vi "write_fifo_resonance_toggle_and_FF_FB.vi"(5 "enable fly-back reversion?":bool, 7 "fly-back?":bool, 8 "pixel finished?":bool, 9 "mark fly-back":bool=TRUE, 11 "integration cluster in":T1) -> (0 "FIFO overflow out":bool, 3 "integration cluster out":T1)   [LabVIEW 2010]
uses:
  integration_cluster.ctl
  <vilib>/rvi/DataTransferAndStorage/Container/XNode/niFpgaContainer.xnode
  <vilib>/rvi/DataTransferAndStorage/Container/Common/niFpgaContainerMethod.ctl
  <vilib>/rvi/DataTransferAndStorage/Container/Common/niFpgaTransferTypeControl.ctl
  <vilib>/rvi/Memory/Memory_Emulation/nirvimemoryEmulationManagerCache_GetValue.vi
  <vilib>/rvi/DataTransferAndStorage/Container/Common/niFpgaContainerGetUniqueNameForEmu.vi
  <vilib>/rvi/Memory/Memory_Emulation/nirvimemoryEmulationManagerCache_InsertValue.vi
  <vilib>/Utility/error.llb/Clear Errors.vi
  <vilib>/rvi/Memory/Memory_Emulation/nirvimemoryEmulationManagerCache_SetValue.vi
  <vilib>/rvi/interface/RandomDataEmulation/nirviRandomDataFPGAFIFO.vi
  <vilib>/rvi/interface/RandomDataEmulation/niFpgaRandomDataHandleErrors.vi
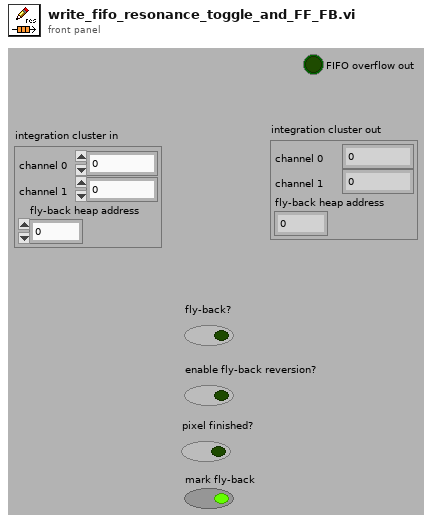
[diagram p1: front panel]
types:
  T1 = typedef "integration_cluster.ctl" = cluster{"channel 0":u32, "channel 1":u32, "fly-back heap address":u32}
  T2 = typedef "niFpgaContainerMethod.ctl" = enum16{"<none>", "write", "read", "clear", "getNumberOfElementsToWrite", "getNumberOfElementsToRead", "enable", "disable", "flushAndDisable", "getStreamState", "readA", "readB", "dramWrite", "dramWriteWithByteEnables", "dramRequestData", "dramRetrieveData"}
  T3 = typedef "niFpgaTransferTypeControl.ctl" = enum16{"Target-Scoped", "Host to Target - DMA", "Target to Host - DMA", "Peer to Peer Reader", "Peer to Peer Writer", "Bidirectional"}
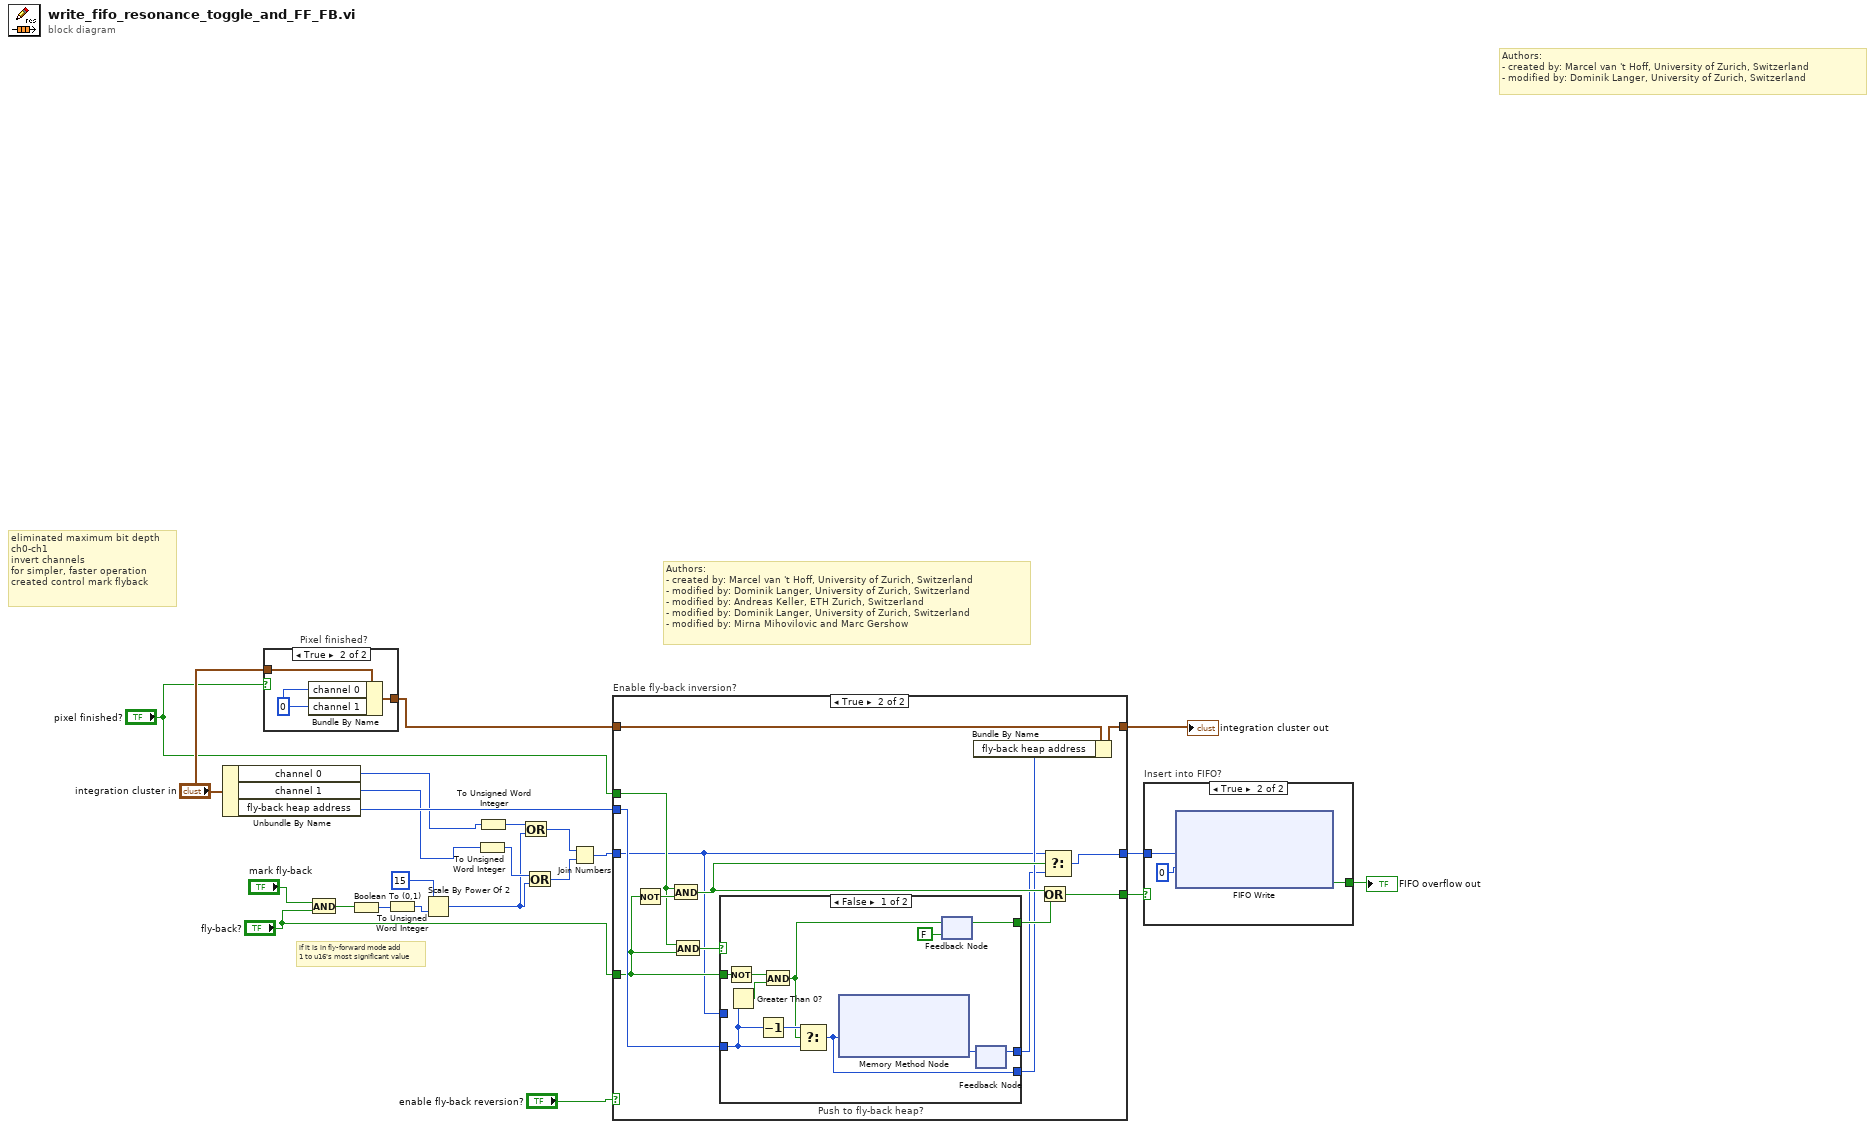
[diagram p0: block diagram]
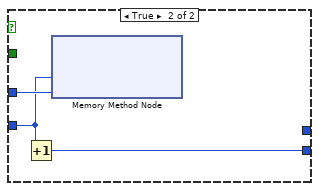
[diagram p4: hidden frame]
diagram:
  # "eliminated maximum bit depth\nch0-ch1\ninvert channels\nfor simpler, faster operation\ncreated control mark flyback"
  # "if it is in fly-forward mode add \n1 to u16's most significant value"
  # "Authors: \n- created by: Marcel van 't Hoff, University of Zurich, Switzerland\n- modified by: Dominik Langer, University of Zurich, Switzerland\n- modified by: Andreas Keller, ETH Zurich, Switzerland\n- modified by: Dominik Langer, University of Zurich, Switzerland\n- modified by: Mirna Mihovilovic and Marc Gershow"
  # "Authors: \n- created by: Marcel van 't Hoff, University of Zurich, Switzerland\n- modified by: Dominik Langer, University of Zurich, Switzerland"
  n1 = Unbundle By Name("integration cluster in") -> ("channel 0"=w11:u32, "channel 1"=w10:u32, "fly-back heap address"=w20:u32)
  n2 = case "Pixel finished?" shown="True" "pixel finished?" {
    tunnel: "integration cluster in" -> [w24 w26]
    tunnel: [w24 w25] -> w17
    frame False {
    }
    frame True {
      w27 = u32 0 ("channel 1")
      n3 = Bundle By Name(cluster=w26, "channel 0"=w27, "channel 1"=w27) -> (w25:T1)
    }
  }
  n4 = And(x="mark fly-back", y="fly-back?") -> (x .and. y?=w7:bool)
  n5 = Boolean To (0,1)(Boolean=w7) -> (0, 1=w6:i16)
  n6 = To Unsigned Word Integer(number=w6) -> (unsigned 16bit integer=w5:u16)
  n7 = Scale By Power Of 2(n=15, x=w5) -> (x*2^n=w3:u16)
  n8 = To Unsigned Word Integer(number=w10) -> (unsigned 16bit integer=w13:u16)
  n9 = To Unsigned Word Integer(number=w11) -> (unsigned 16bit integer=w14:u16)
  n10 = Or(x=w14, y=w3) -> (x .or. y?=w2:u16)
  n11 = Or(x=w13, y=w3) -> (x .or. y?=w1:u16)
  n12 = Join Numbers(hi=w2, lo=w1) -> ((hi.lo)=w12:u32)
  n13 = case "Enable fly-back inversion?" shown="True" "enable fly-back reversion?" {
    tunnel: w20 -> [_ w44]
    tunnel: w12 -> [w30 w33]
    tunnel: [w30 w42] -> w22
    tunnel: "pixel finished?" -> [w29 w37]
    tunnel: [w29 w32] -> w19
    tunnel: "fly-back?" -> [_ w39]
    tunnel: w17 -> [w28 w36]
    tunnel: [w28 w34] -> w15
    frame False {
    }
    frame True {
      n14 = Not(x=w39) -> (.not. x?=w43:bool)
      n15 = And(x=w37, y=w43) -> (x .and. y?=w40:bool)
      n16 = And(x=w37, y=w39) -> (x .and. y?=w41:bool)
      n17 = case "Push to fly-back heap?" shown="False" w41 {
        tunnel: w33 -> [_ w184]
        tunnel: [w47 w183] -> w35
        tunnel: w44 -> [w49 w182]
        tunnel: w39 -> [w54 _]
        tunnel: [w51 _] -> w31
        tunnel: [w53 _] -> w38
        frame False {
          n18 = Not(x=w54) -> (.not. x?=w46:bool)
          n19 = Greater Than 0?(x=w49) -> (x > 0?=w55:bool)
          n20 = Decrement(x=w49) -> (x-1=w48:u32)
          n21 = And(x=w46, y=w55) -> (x .and. y?=w45:bool)
          n22 = Select(t=w48, s=w45, f=w49) -> (s? t:f=w47:u32)
          n23 = xnode ("Memory Method Node")("Address"=w47) -> ("Data"=w50:u32)  [unwired: 1 in, 1 out]
          n24 = feedback #1(FALSE) -> (w53:bool)
          n25 = feedback-in #1(w45) -> ()
          n26 = feedback #2() -> (w51:u32)  [unwired: 1 in]
          n27 = feedback-in #2(w50) -> ()
        }
        frame True {
          n28 = Increment(x=w182) -> (x+1=w183:u32)
          n29 = xnode ("Memory Method Node")("Address"=w182, "Data"=w184) -> ()  [unwired: 1 in, 1 out]
        }
      }
      n30 = Bundle By Name(cluster=w36, "fly-back heap address"=w35) -> (w34:T1)
      n31 = Or(x=w40, y=w38) -> (x .or. y?=w32:bool)
      n32 = Select(t=w33, s=w40, f=w31) -> (s? t:f=w42:u32)
    }
  }
  "integration cluster out" <- w15
  n33 = case "Insert into FIFO?" shown="True" w19 {
    tunnel: [_ w312] -> w23
    tunnel: w22 -> [_ w310]
    frame False {
    }
    frame True {
      n34 = xnode ("FIFO Write")("Element"=w310, "Timeout"=0) -> ("Timed Out?"=w312:bool)  [unwired: 1 in, 1 out]
    }
  }
  "FIFO overflow out" <- w23
